vi "weblink destroy.vi"(0 "Link Picture Ref (NULL)":refnum<vi>) -> ()   [LabVIEW 2011]
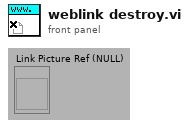
[diagram p1: front panel]
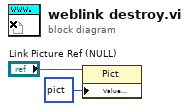
[diagram p0: block diagram]
diagram:
  n1 = property class="Pict"(reference="Link Picture Ref (NULL)", "Value (Signaling)"=picture data[5B]) -> ()  [unwired: 1 in, 2 out]
